vi "tdms test.vi"(11 "logrotate_options":T1={"max file size (bytes)"=10000, "rotate count"=5, "max age (days)"=3.0, "No archive dir"=FALSE, "Archive dir"=path ""}) -> (0 "error out":errorcluster, 3 "found?":bool)   [LabVIEW 2015, in "tdms logger tests.lvlib"]
uses:
  tdms logger tests.lvlib
  <vilib>/NI/LogRotate/options.ctl
  configuration/TDMS datalogger configuration.lvclass
  execution/TDMS datalogger runtime.lvclass
  <vilib>/NI/Tag Bus Module Framework/channel/channel classification.ctl
  <vilib>/NI/Tag Bus/tag/Data Type.ctl
  <vilib>/Platform/TimedLoop/XDataNode/timing_clust.ctl
  <vilib>/Platform/TimedLoop/XDataNode/nitl_modes.ctl
  <vilib>/Platform/TimedLoop/XDataNode/wakeup.ctl
  <vilib>/NI/Tag Bus/tag/tag descriptor.lvclass/tag descriptor.ctl
  configuration/TDMS datalogger configuration.lvclass/TDMS datalogger configuration.ctl
  <vilib>/NI/Tag Bus/table/data polymorphs/write one/write Boolean.vi
  configuration/Write Path.vi
  configuration/Write queue size.vi
  configuration/Write scans per write.vi
  configuration/Write backup directory.vi
  configuration/Write add enable channel.vi
  configuration/Write log name.vi
  configuration/Write logrotate_options.vi
  <vilib>/platform/TimedLoop/XDataNode/XDataNode.xnode
  <vilib>/NI/Tag Bus Module Framework/channel/TBM channel.lvclass
  <vilib>/NI/Tag Bus/tag/tag descriptor.lvclass
  <vilib>/NI/Tag Bus/table/data table.lvlib
  <vilib>/Platform/TimedLoop/XDataNode/XDNodeRunTimeDep.lvlib
  <vilib>/Utility/RT CPU pool selections.ctl
  <vilib>/NI/Configuration Framework/serializable configuration/NISE_CEF_serializable configuration.lvclass
  <vilib>/NI/LogRotate/LogRotate.lvclass
panel:
  in  "iterations":i32=1000
  in  "scans per write":i32=20
  in  "queue size":i32=20
  out "max":dbl
  out "min":dbl
  in  "enable state":bool=TRUE
  in  "stop":bool
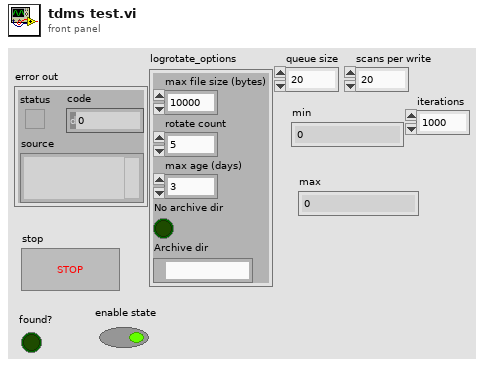
[diagram p1: front panel]
types:
  T1 = typedef "LogRotate.lvclass/options.ctl" = cluster{"max file size (bytes)":i64, "rotate count":u32, "max age (days)":dbl, "No archive dir":bool, "Archive dir":path}
  T2 = typedef "tag bus.lvlib/tag descriptor.lvclass/Data Type.ctl" = enum16{"Double", "Single", "I64", "I32", "I16", "I8", "U64", "U32", "U16", "U8", "Boolean", "String", "Array of Double", "Array of Single", "Array of I64", "Array of I32", "Array of I16", "Array of I8", "Array of U64", "Array of U32", "Array of U16", "Array of U8", "Array of Boolean", "Array of String"}
  T3 = typedef "TBM channel.lvclass/channel classification.ctl" = enum16{"input data", "output data", "processing parameter", "processing result"}
  T4 = typedef "NI_Real-Time Target Support.lvlib/RT CPU pool selections.ctl" = enum16{"System & Timed Structures", "System", "Timed Structures", "Reserved"}
  T5 = typedef "TBM channel.lvclass/data tables.ctl" = cluster{"input data":T6, "processing parameter":T6, "processing result":T6, "output data":T6}
  T6 = typedef "tag bus.lvlib/dictionary table pair.ctl" = cluster{"data dictionary":refnum<class "data dictionary.lvclass">, "data table":T7}
  T7 = typedef "tag bus.lvlib/data table.lvlib/data table.ctl" = cluster{"Double":dbl[], "Single":sgl[], "I64":i64[], "I32":i32[], "I16":i16[], "I8":i8[], "U64":u64[], "U32":u32[], "U16":u16[], "U8":u8[], "Boolean":bool[], "String":string[], "Array of Double":cluster{"DBL Array":dbl[]}[], "Array of Single":cluster{"SGL Array":sgl[]}[], "Array of I64":cluster{"I64 Array":i64[]}[], "Array of I32":cluster{"I32 Array":i32[]}[], "Array of I16":cluster{"I16 Array":i16[]}[], "Array of I8":cluster{"I8 Array":i8[]}[], "Array of U64":cluster{"U64 Array":u64[]}[], "Array of U32":cluster{"U32 Array":u32[]}[], "Array of U16":cluster{"U16 Array":u16[]}[], "Array of U8":cluster{"U8 Array":u8[]}[], "Array of Boolean":cluster{"Boolean Array":bool[]}[], "Array of String":cluster{"String Array":string[]}[]}
  T8 = typedef "XDNodeRunTimeDep.lvlib/timing_clust.ctl" = cluster{"Expected End [f-1]":u64, "Actual End [f-1]":u64, "Finished Late? [f-1]":bool, "Expected End [i-1]":u64, "Actual End [i-1]":u64, "Finished Late? [i-1]":bool, "Expected Start [i]":u64, "Actual Start [i]":u64, "Expected Start [f]":u64, "Actual Start [f]":u64, "Source Name":string, "Structure Name":string, "Period":i64, "Deadline":i64, "Offset":i64, "Start":i64, "Priority":i32, "Timeout":i32, "Mode":T9, "Wakeup Reason":T10, "Error":errorcluster, "Source Type":string, "Secondary Source Type":string, "Global End Time":u64, "Global Start Time":u64, "Frame Duration":u64, "Iteration Duration":u64, "Assigned CPU":i32, "I/O Scan Engine Mode":u32}
  T9 = typedef "XDNodeRunTimeDep.lvlib/nitl_modes.ctl" = enum32{"No Change", "Process missed periods, maintain original phase", "Discard missed periods, maintain original phase", "Process missed periods, ignore original phase", "Discard missed periods, ignore original phase"}
  T10 = typedef "XDNodeRunTimeDep.lvlib/wakeup.ctl" = enum32{"Normal", "Aborted", "Asynchronous wakeup", "Timing source error", "Timed loop error", "Timeout"}
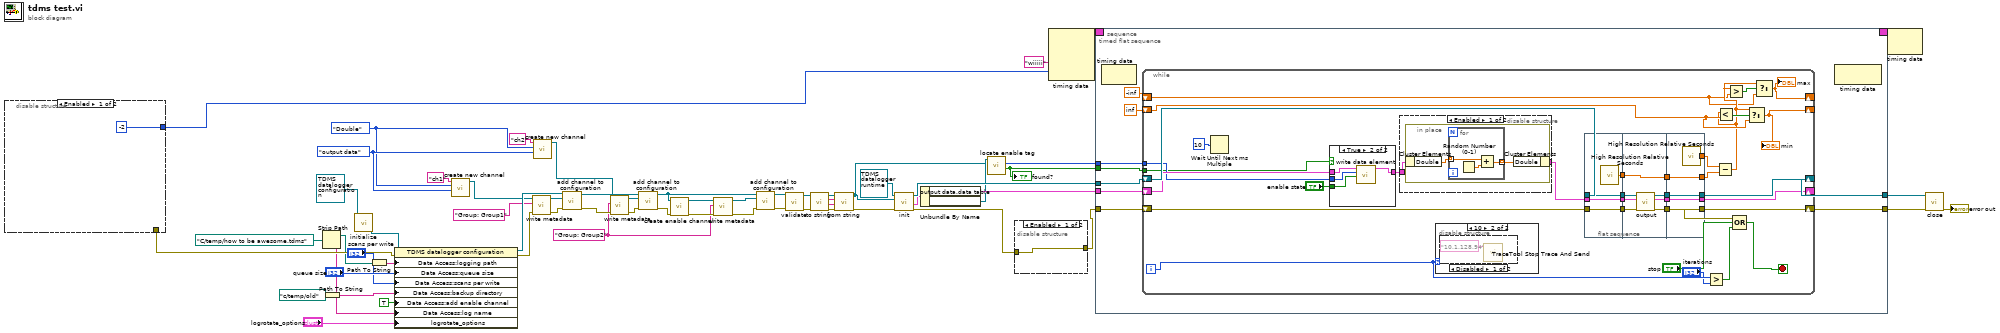
[diagram p0: block diagram]
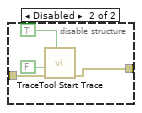
[diagram p2: hidden frame]
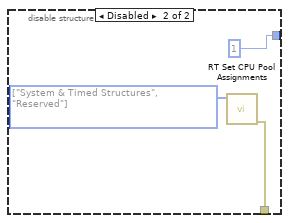
[diagram p3: hidden frame]
diagram:
  w1 = "Group: Group2" ("metadata")
  w45 = Data_Type."Double" ("data type")
  w46 = channel_classification."output data" ("channel classification")
  n1 = disable-structure shown="Enabled" {
    disable-tunnel: [_ w64] -> w33
    disable-tunnel: [-2 ("Processor") 1 ("Processor")] -> w32
    frame Enabled {
    }
    frame Disabled {
      w65 = T4[] [enum."System & Timed Structures", enum."Reserved"] items=["System & Timed Structures", "System", "Timed Structures", "Reserved"] ("CPU pools")
      n2 = call <vilib>:"RT Set CPU Pool Assignments.vi"("CPU pools"=w65) -> ("error out"=w64:errorcluster)  [unwired: 7 in, 3 out]
    }
  }
  n3 = Strip Path(path=path "C:/temp/how to be awesome.tdms" ("output file path")) -> (stripped path=w19:path, name=w17:string)
  n4 = Path To String(path=path "c:/temp/old" ("output file path")) -> (string=w16:string)
  n5 = call <vilib>:"initialize.vi"("configuration in"=refnum<class "TDMS datalogger configuration.lvclass"> refnum ("TDMS datalogger configuration")) -> ("configuration out"=w21:refnum<class "TDMS datalogger configuration.lvclass">)  [unwired: 8 in, 2 out]
  n6 = Path To String(path=w19) -> (string=w18:string)
  n7 = property class="TDMS datalogger configuration"(reference=w21, error in=w33, "Data Access:logging path"=w18, "Data Access:queue size"="queue size", "Data Access:scans per write"="scans per write", "Data Access:backup directory"=w16, "Data Access:add enable channel"=TRUE ("add enable channel"), "Data Access:log name"=w17, "logrotate_options"="logrotate_options") -> (reference out=w25:refnum<class "TDMS datalogger configuration.lvclass">, error out=w7:errorcluster)
  n8 = call <vilib>:"create new channel.vi"("channel classification"=w46, "data type"=w45, "channel name"="ch1") -> ("channel"=w10:refnum<class "TBM channel.lvclass">)  [unwired: 8 in]
  n9 = call <vilib>:"write metadata.vi"("error in"=w7, "metadata"="Group: Group1", "system tag in"=w10) -> ("error out"=w6:errorcluster, "system tag out"=w11:refnum<class "TBM channel.lvclass">)  [unwired: 7 in]
  n10 = call <vilib>:"create new channel.vi"("channel classification"=w46, "data type"=w45, "channel name"="ch2") -> ("channel"=w14:refnum<class "TBM channel.lvclass">)  [unwired: 8 in]
  n11 = call "add channel to configuration.vi"("error in"=w6, "TBM channel in"=w11, "TDMS datalogger configuration in"=w25) -> ("error out"=w9:errorcluster, "TDMS datalogger configuration out"=w26:refnum<class "TDMS datalogger configuration.lvclass">)  [unwired: 7 in]
  n12 = call <vilib>:"write metadata.vi"("error in"=w9, "metadata"=w1, "system tag in"=w14) -> ("error out"=w8:errorcluster, "system tag out"=w13:refnum<class "TBM channel.lvclass">)  [unwired: 7 in]
  n13 = call "add channel to configuration.vi"("error in"=w8, "TBM channel in"=w13, "TDMS datalogger configuration in"=w26) -> ("error out"=w24:errorcluster, "TDMS datalogger configuration out"=w23:refnum<class "TDMS datalogger configuration.lvclass">)  [unwired: 7 in]
  n14 = call "create enable channel.vi"("error in"=w24, "TDMS datalogger configuration"=w23) -> ("error out"=w3:errorcluster, "enable channel"=w5:refnum<class "TBM channel.lvclass">)  [unwired: 7 in, 1 out]
  n15 = call <vilib>:"write metadata.vi"("error in"=w3, "metadata"=w1, "system tag in"=w5) -> ("error out"=w2:errorcluster, "system tag out"=w4:refnum<class "TBM channel.lvclass">)  [unwired: 7 in]
  n16 = call "add channel to configuration.vi"("error in"=w2, "TBM channel in"=w4, "TDMS datalogger configuration in"=w23) -> ("error out"=w28:errorcluster, "TDMS datalogger configuration out"=w27:refnum<class "TDMS datalogger configuration.lvclass">)  [unwired: 7 in]
  n17 = call-dynamic "validate.vi"("error in"=w28, "TDMS datalogger configuration in"=w27) -> ("error out"=w61:errorcluster, "TDMS datalogger configuration out"=w60:refnum<class "TDMS datalogger configuration.lvclass">)  [unwired: 8 in]
  n18 = call-dynamic "to string.vi"("error in"=w61, "TDMS datalogger configuration in"=w60) -> ("error out"=w58:errorcluster, "data"=w57:string, "version"=w56:string, "TDMS datalogger configuration out"=w59:refnum<class "TDMS datalogger configuration.lvclass">)  [unwired: 6 in]
  n19 = call-dynamic "from string.vi"("error in"=w58, "data"=w57, "version"=w56, "TDMS datalogger configuration in"=w59) -> ("error out"=w55:errorcluster, "TDMS datalogger configuration out"=w22:refnum<class "TDMS datalogger configuration.lvclass">)  [unwired: 6 in]
  n20 = call-dynamic "init.vi"("error in"=w55, "TBM module configuration in"=w22, "TDMS datalogger runtime in"=refnum<class "TDMS datalogger runtime.lvclass"> refnum ("TDMS datalogger runtime")) -> ("error out"=w31:errorcluster, "data allocations"=w47:T5, "TDMS datalogger runtime out"=w54:refnum<class "TDMS datalogger runtime.lvclass">)  [unwired: 5 in, 1 out]
  n21 = Unbundle By Name(w47) -> ("output data.data table"=w53:T7, "output data.data dictionary"=w38:refnum<class "data dictionary.lvclass">)
  n22 = call "locate enable tag.vi"("TDMS datalogger configuration"=w22, "data dictionary in"=w38) -> ("found?"=w36:bool, "index"=w37:i32)  [unwired: 7 in, 1 out]
  "found?" <- w36
  n23 = disable-structure shown="Enabled" {
    disable-tunnel: [w66 w69] -> w30
    disable-tunnel: w31 -> [w66 w70]
    frame Enabled {
    }
    frame Disabled {
      n24 = call <vilib>:"TraceTool Start Trace.vi"("Detailed Tracing? (F)"=TRUE, "error in (no error)"=w70, "VI Tracing? (T)"=FALSE) -> ("error out"=w69:errorcluster)  [unwired: 7 in, 1 out]
    }
  }
  n25 = node-c288("wiiiii" ("Structure Name"), w32) -> (w35:T8)  [unwired: 2 in]
  n26 = timed-sequence {
    timing: w35 -> [_]
    timing-out: [_] -> w34
    tunnel: w54 -> [w77]
    tunnel: w30 -> [w76]
    tunnel: w53 -> [w75]
    tunnel: [w74] -> w52
    tunnel: [w73] -> w51
    tunnel: w37 -> [w72]
    tunnel: w36 -> [w71]
    n27 = timed-flat-sequence {
      tunnel: w77 -> [w86]
      tunnel: w76 -> [w85]
      tunnel: w75 -> [w84]
      tunnel: [w83] -> w74
      tunnel: [w82] -> w73
      tunnel: w72 -> [w81]
      tunnel: w71 -> [w80]
      n28 = node-c288() -> ()  [unwired: 1 in, 1 out]
      n29 = while {
        shift-right: [w108] -> w82
        shift-left: w85 -> [w119]
        shift-right: [w118] -> w83
        shift-left: w86 -> [w120]
        shift-right: [w116] -> _
        shift-left: w84 -> [w113]
        tunnel: w81 -> [w111]
        tunnel: w80 -> [w110]
        shift-right: [w91] -> _
        shift-left: -inf -> [w93]
        shift-right: [w92] -> _
        shift-left: inf -> [w95]
        i -> [w89]
        stop <- w109 stop-if-true
        n30 = Wait Until Next ms Multiple(millisecond multiple=u32 10) -> ()  [unwired: 1 out]
        n31 = case shown="True" w110 {
          tunnel: w113 -> [w121 w125]
          tunnel: [w121 w124] -> w112
          tunnel: w111 -> [_ w123]
          tunnel: "enable state" -> [_ w122]
          frame False {
          }
          frame True {
            n32 = call-poly <vilib>:"write data element.vi"("value"=w122, "index"=w123, "data table in"=w125) -> ("data table out"=w124:T7)  [unwired: 8 in]
          }
        }
        n33 = disable-structure shown="Enabled" {
          disable-tunnel: [w144 w150] -> w117
          disable-tunnel: w112 -> [w143 w150]
          frame Enabled {
            n34 = in-place {
              n35 = in-place-cluster #1(w143) -> ("Double"=w146:dbl[])
              n36 = for {
                tunnel: w146 -> [w149] mode=indexing
                tunnel: [w148] -> w145 mode=indexing
                n37 = Random Number (0-1)() -> (number: 0 to 1=w147:dbl)
                n38 = Add(x=w149, y=w147) -> (x+y=w148:dbl)
              }
              n39 = in-place-cluster #1("Double"=w145) -> (w144:T7)
            }
          }
          frame Disabled {
          }
        }
        n40 = case shown="10" w89 {
          frame 0, Default {
          }
          frame 10 {
            n41 = disable-structure shown="Disabled" {
              frame Disabled {
                n42 = call <vilib>:"TraceTool Stop Trace And Send.vi"("Trace Host Network Address"="10.1.128.94") -> ()  [unwired: 10 in, 1 out]
              }
              frame Enabled {
              }
            }
          }
        }
        n43 = flat-sequence {
          tunnel: w117 -> [w128]
          tunnel: w119 -> [w129]
          tunnel: w120 -> [w130]
          tunnel: [w130] -> w104
          tunnel: [w129] -> w103
          tunnel: [w128] -> w102
          tunnel: [w127] -> w100
          tunnel: [w135] -> w107
          tunnel: [w133] -> w106
          tunnel: [w132] -> w105
          tunnel: w104 -> [w137]
          tunnel: w103 -> [w136]
          tunnel: w102 -> [w134]
          tunnel: [w131] -> w101
          tunnel: w100 -> [w131]
          tunnel: [w140] -> w108
          tunnel: [w141] -> w116
          tunnel: [w142] -> w118
          tunnel: w107 -> [w142]
          tunnel: w106 -> [w141]
          tunnel: w105 -> [w140]
          tunnel: [w139] -> w99
          tunnel: w101 -> [w139]
          tunnel: [w138] -> w98
          frame #0 {
            n44 = call <vilib>:"High Resolution Relative Seconds.vi"() -> ("relative seconds"=w127:dbl)
          }
          frame #1 {
            n45 = call-dynamic "output.vi"("error in"=w136, "data table in"=w134, "TDMS datalogger runtime in"=w137) -> ("error out"=w132:errorcluster, "data table out"=w133:T7, "TDMS datalogger runtime out"=w135:refnum<class "TDMS datalogger runtime.lvclass">)  [unwired: 6 in]
          }
          frame #2 {
            n46 = call <vilib>:"High Resolution Relative Seconds.vi"() -> ("relative seconds"=w138:dbl)
          }
        }
        n47 = Greater?(x=w89, y="iterations") -> (0:w87:bool)
        n48 = Subtract(x=w98, y=w99) -> (x-y=w94:dbl)
        n49 = Less?(x=w94, y=w95) -> (x < y?=w96:bool)
        n50 = Greater?(x=w94, y=w93) -> (0:w97:bool)
        n51 = Compound Arithmetic op=OR(w108, "stop", w87) -> (w109:bool)
        n52 = Select(t=w94, s=w96, f=w95) -> (s? t:f=w92:dbl)
        "min" <- w92
        n53 = Select(t=w94, s=w97, f=w93) -> (s? t:f=w91:dbl)
        "max" <- w91
      }
      n54 = node-c288() -> ()  [unwired: 1 in, 1 out]
    }
  }
  n55 = node-c288(w34) -> ()  [unwired: 1 out]
  n56 = call-dynamic "close.vi"("error in"=w51, "TDMS datalogger runtime in"=w52) -> ("error out"=→"error out":errorcluster)  [unwired: 9 in]
